vi "Main UI.vi"(11 "App in":refnum<class "App.lvclass">) -> (3 "App":refnum<class "App.lvclass">)   [LabVIEW 2020, in "App.lvclass"]
uses:
  App.lvclass
  App.lvclass/App.ctl
  Blueprint Qty.ctl
  Blueprint/Blueprint.lvclass
  Item Summary/Item Summary.lvclass
  C:/Program Files (x86)/National Instruments/LabVIEW 2020/vi.lib/IlluminatedG/IG OOPanel/OOPanel/ArrayPanel/ArrayPanel.lvclass
  BP Summary/BP Summary.lvclass
  <vilib>/IlluminatedG/IG OOPanel/OOPanel/ArrayManager/ArrayManager.lvclass
panel:
  in  "New Button":bool
  in  "Add Button":bool
  # "Good Company Blueprints"
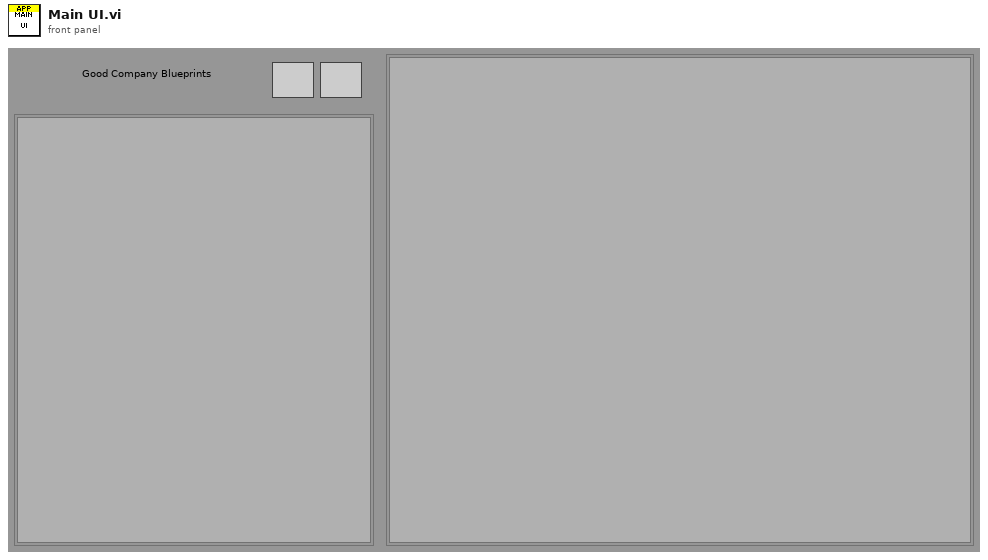
[diagram p1: front panel]
types:
  T1 = typedef "App.lvclass/Blueprint Qty.ctl" = cluster{"Blueprint":refnum<class "Blueprint.lvclass">, "Qty":dbl}
  T2 = typedef "Item.lvclass/Ingredient.ctl" = cluster{"Item":refnum<class "Item.lvclass">, "Qty":dbl}
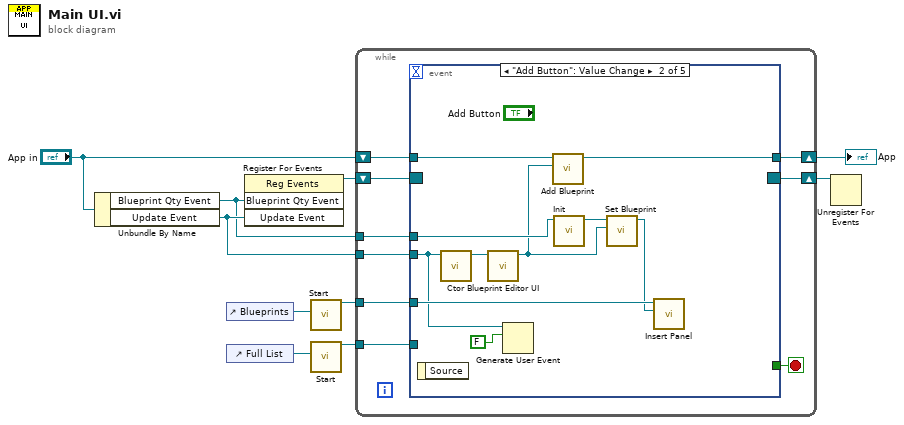
[diagram p0: block diagram]
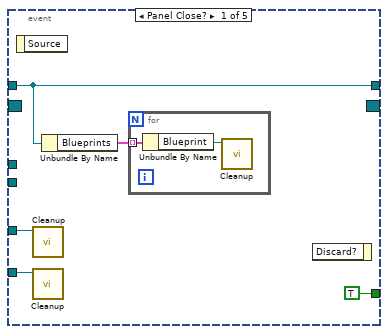
[diagram p2: hidden frame]
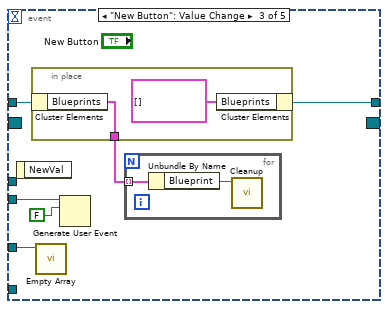
[diagram p3: hidden frame]
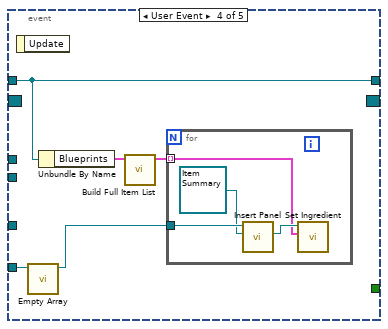
[diagram p4: hidden frame]
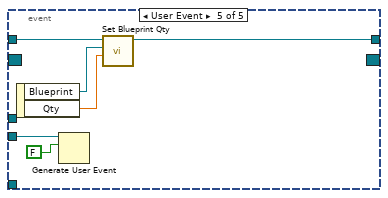
[diagram p5: hidden frame]
diagram:
  n1 = Unbundle By Name("App in") -> ("Blueprint Qty Event"=w2:refnum<user-event>, "Update Event"=w5:refnum<user-event>)
  n2 = control-ref of="Blueprints"() -> (w10:refnum<vi>)
  n3 = control-ref of="Full List"() -> (w9:refnum<vi>)
  n4 = register-events(w2, w5) -> (reference out=w6:refnum<event-registration>)  [unwired: 2 in, 1 out]
  n5 = call <vilib>:"Start.vi"("Container"=w10) -> ("ArrayManager out"=w8:refnum<class "ArrayManager.lvclass">)  [unwired: 9 in, 1 out]
  n6 = call <vilib>:"Start.vi"("Container"=w9) -> ("ArrayManager out"=w7:refnum<class "ArrayManager.lvclass">)  [unwired: 9 in, 1 out]
  n7 = while {
    tunnel: w8 -> [w19]
    tunnel: w7 -> [w18]
    shift-right: [w15] -> w1
    shift-left: w6 -> [w16]
    tunnel: w5 -> [w14]
    shift-right: [w12] -> w3
    shift-left: "App in" -> [w13]
    tunnel: w2 -> [w11]
    stop <- w17 stop-if-true
    n8 = event shown="[1] \"Add Button\": Value Change" {
      selector: w16 -> [_ _ _ _ _]
      dyn-events: [_ _ _ _ _] -> w15
      timeout: _ -> [_ _ _ _ _]
      tunnel: w19 -> [w24 w35 w40 _ _]
      tunnel: w18 -> [w23 _ _ w51 _]
      tunnel: [TRUE ("Discard?") _ _ _ _] -> w17
      tunnel: w14 -> [_ w32 w42 _ w61]
      tunnel: w13 -> [w20 w33 w39 w50 w59]
      tunnel: [w20 w30 w37 w50 w56] -> w12
      tunnel: w11 -> [_ w29 _ _ _]
      event Panel Close? {
        n9 = event-data() -> ()  [unwired: 1 in, 1 out]
        n10 = call <vilib>:"Cleanup.vi"("PanelArray in"=w24) -> ()  [unwired: 10 in, 1 out]
        n11 = call <vilib>:"Cleanup.vi"("PanelArray in"=w23) -> ()  [unwired: 10 in, 1 out]
        n12 = Unbundle By Name(w20) -> ("Blueprints"=w21:T1[])
        n13 = for {
          tunnel: w21 -> [w26] mode=indexing
          n14 = Unbundle By Name(w26) -> ("Blueprint"=w25:refnum<class "Blueprint.lvclass">)
          n15 = call <vilib>:"Cleanup.vi"("Blueprint in"=w25) -> ()  [unwired: 10 in, 1 out]
        }
        n16 = event-data() -> ()  [unwired: 2 in, 1 out]
      }
      event "Add Button": Value Change {
        n17 = event-data() -> ()  [unwired: 1 in, 1 out]
        n18 = call "Ctor.vi"("Update Event"=w32) -> ("Blueprint out"=w36:refnum<class "Blueprint.lvclass">)  [unwired: 9 in, 1 out]
        n19 = call "Blueprint Editor UI.vi"("Blueprint in"=w36) -> ("Blueprint"=w27:refnum<class "Blueprint.lvclass">)  [unwired: 10 in]
        n20 = Generate User Event(user event=w32, event data cluster=FALSE ("event data")) -> ()  [unwired: 2 in, 2 out]
        n21 = call "Add Blueprint.vi"("Blueprint"=w27, "App in"=w33) -> ("App out"=w30:refnum<class "App.lvclass">)  [unwired: 8 in, 1 out]
        n22 = call "Init.vi"("Blueprint Qty Event"=w29) -> ("BP Summary out"=w28:refnum<class "BP Summary.lvclass">)  [unwired: 9 in, 1 out]
        n23 = call "Set Blueprint.vi"("Blueprint"=w27, "BP Summary in"=w28) -> ("BP Summary out"=w34:refnum<class "BP Summary.lvclass">)  [unwired: 8 in, 1 out]
        n24 = call <vilib>:"Insert Panel.vi"("Panel/Type"=w34, "PanelArray in"=w35) -> ()  [unwired: 7 in, 3 out]
      }
      event "New Button": Value Change {
        n25 = event-data() -> ()  [unwired: 1 in, 1 out]
        n26 = in-place {
          in-place-border: [w45] -> w38
          n27 = in-place-cluster #1(w39) -> ("Blueprints"=w45:T1[])
          n28 = in-place-cluster #1("Blueprints"=T1[] []) -> (w37:refnum<class "App.lvclass">)
        }
        n29 = call <vilib>:"Empty Array.vi"("ArrayManager in"=w40) -> ()  [unwired: 9 in, 2 out]
        n30 = Generate User Event(user event=w42, event data cluster=FALSE ("event data")) -> ()  [unwired: 2 in, 2 out]
        n31 = for {
          tunnel: w38 -> [w44] mode=indexing
          n32 = Unbundle By Name(w44) -> ("Blueprint"=w43:refnum<class "Blueprint.lvclass">)
          n33 = call <vilib>:"Cleanup.vi"("Blueprint in"=w43) -> ()  [unwired: 10 in, 1 out]
        }
      }
      event User Event {
        n34 = event-data() -> ()  [unwired: 1 in, 1 out]
        n35 = call <vilib>:"Empty Array.vi"("ArrayManager in"=w51) -> ("ArrayManager out"=w47:refnum<class "ArrayManager.lvclass">)  [unwired: 9 in, 1 out]
        n36 = Unbundle By Name(w50) -> ("Blueprints"=w49:T1[])
        n37 = call "Build Full Item List.vi"("Components"=w49) -> ("Total Ingredients"=w48:T2[])  [unwired: 10 in]
        n38 = for {
          tunnel: w47 -> [w55]
          tunnel: w48 -> [w52] mode=indexing
          n39 = call <vilib>:"Insert Panel.vi"("Panel/Type"=refnum<class "Item Summary.lvclass"> refnum ("Item Summary.lvclass"), "PanelArray in"=w55) -> ("Panel"=w53:refnum<class "Item Summary.lvclass">)  [unwired: 7 in, 2 out]
          n40 = call "Set Ingredient.vi"("Ingredient"=w52, "Item Summary in"=w53) -> ()  [unwired: 8 in, 2 out]
        }
      }
      event User Event {
        n41 = event-data() -> ("Blueprint"=w58:refnum<class "Blueprint.lvclass">, "Qty"=w57:dbl)  [unwired: 1 in]
        n42 = Generate User Event(user event=w61, event data cluster=FALSE ("event data")) -> ()  [unwired: 2 in, 2 out]
        n43 = call "Set Blueprint Qty.vi"("Qty"=w57, "Blueprint"=w58, "App in"=w59) -> ("App out"=w56:refnum<class "App.lvclass">)  [unwired: 7 in, 1 out]
      }
    }
  }
  "App" <- w3
  n44 = Unregister For Events(event registration refnum=w1) -> ()  [unwired: 1 in, 1 out]
